vi "ESP_Full_State_Test_UDP.vi"() -> ()   [LabVIEW 2021]
panel:
  out "output array":sgl[][](array[numeric])
  out "Waveform Chart 2":sgl[][](graph)
  out "Waveform Chart":sgl[](graph)
  out "Close UPD":bool=TRUE
  out "Data":dbl[](array[numeric])
  out "Stream on? UDP":string
  # "Sampling rate is 225 Hz, please use the Setup software to change the rate"
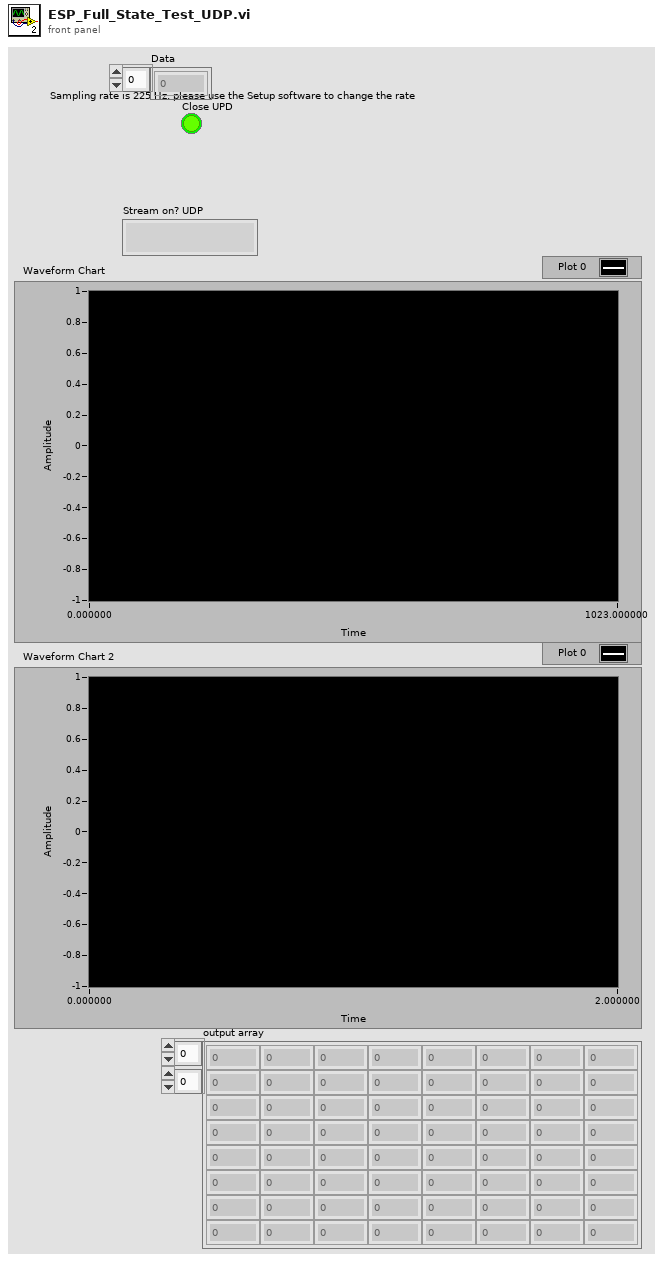
[diagram p1: front panel]
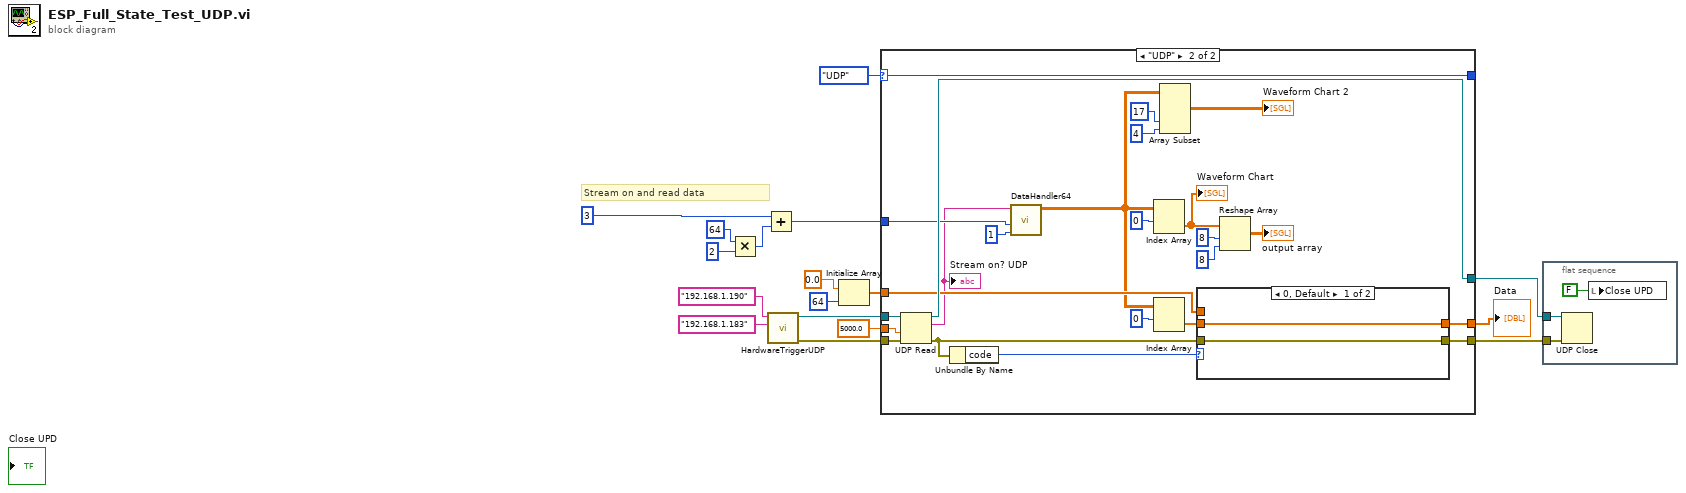
[diagram p0: block diagram]
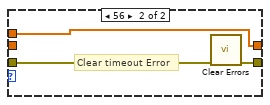
[diagram p3: hidden frame]
diagram:
  # "Stream on and read data"
  n1 = Multiply(x=64, y=2) -> (x*y=w10:i32)
  n2 = Add(x=3, y=w10) -> (x+y=w7:i32)
  n3 = call "HardwareTriggerUDP.vi"("Local IP address"="192.168.1.183", "Remote IP address"="192.168.1.190") -> ("error out"=w6:errorcluster, "connection ID out"=w12:refnum<k16>)  [unwired: 8 in]
  n4 = Initialize Array(0.0, 64) -> (w15:dbl[])
  n5 = case shown="\"UDP\"" enum16{"Off", "UDP"}."UDP" {
    selector: enum16{"Off", "UDP"}."UDP" -> [w21 w44]
    tunnel: w7 -> [_ w32]
    tunnel: w6 -> [w20 w45]
    tunnel: [w20 w40] -> w2
    tunnel: [w21 w44] -> _
    tunnel: [w18 w36] -> w14
    tunnel: 5000.0 -> [_ w37]
    tunnel: w12 -> [w19 w39]
    tunnel: [w19 w38] -> w13
    tunnel: w15 -> [w18 w35]
    frame "Off", Default {
    }
    frame "UDP" {
      n6 = UDP Read(connection ID=w39, timeout ms (25000)=w37, 8:w45) -> (data out=w31:string, error out=w41:errorcluster, 3:w38:refnum<k16>)  [unwired: 1 in, 2 out]
      "Stream on? UDP" <- w31
      n7 = Unbundle By Name(w41) -> ("code"=w42:i32)
      n8 = call "DataHandler64.vi"("Data Cycles Per Buffer"=1, "Rx Packet Byte size"=w32, "data out"=w31) -> ("Data"=w22:sgl[][])  [unwired: 2 in, 4 out]
      n9 = Index Array(array=w22, index (row)=0 ("Channel")) -> (element=w24:sgl[])  [unwired: 1 in]
      "Waveform Chart" <- w24
      n10 = Index Array(array=w22, index (row)=0 ("Data Cycles Per Buffer")) -> (element=w34:sgl[])  [unwired: 1 in]
      n11 = Array Subset(array=w22, index (col)=17 ("index"), length (col)=4 ("length")) -> (→"Waveform Chart 2":sgl[][])  [unwired: 2 in]
      n12 = case shown="0, Default" w42 {
        tunnel: w41 -> [w47 w50]
        tunnel: [w47 w49] -> w40
        tunnel: w34 -> [w46 _]
        tunnel: [w46 w48] -> w36
        tunnel: w35 -> [_ w48]
        frame 0, Default {
        }
        frame 56 {
          # "Clear timeout Error"
          n13 = call <vilib>:"Clear Errors.vi"("error in (no error)"=w50) -> ("error out"=w49:errorcluster)  [unwired: 5 in, 1 out]
        }
      }
      n14 = Reshape Array(w24, 8 ("dimension size"), 8 ("dimension size")) -> (→"output array":sgl[][])
    }
  }
  "Data" <- w14
  n15 = flat-sequence {
    tunnel: w13 -> [w52]
    tunnel: w2 -> [w51]
    frame #0 {
      n16 = UDP Close(connection ID=w52, 8:w51) -> ()  [unwired: 2 out]
      n17 = local write "Close UPD"(FALSE) -> ()
    }
  }
